vi "OpenConfigFile.vi"(8 "error in (no error)":errorcluster, 11 "GRMActor in":refnum<class "GenericController.lvclass">) -> (0 "error out":errorcluster, 2 "refnum":T1, 3 "GRMActor out":refnum<class "GenericController.lvclass">)   [LabVIEW 2020, in "GenericController.lvlib" / "GenericController.lvclass"]
uses:
  GenericController.lvclass
  <vilib>/Utility/config.llb/Config Data RefNum.ctl
  GenericController.lvclass/GenericController.ctl
  <vilib>/Utility/config.llb/NI_LVConfig.lvlib
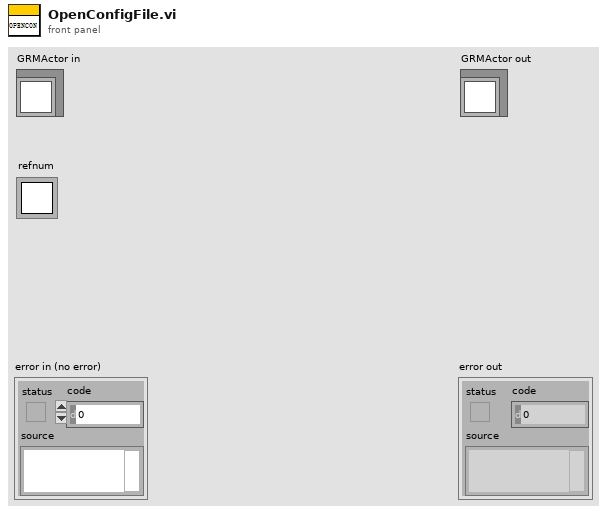
[diagram p1: front panel]
types:
  T1 = typedef "NI_LVConfig.lvlib/Config Data RefNum.ctl" = refnum<k1>
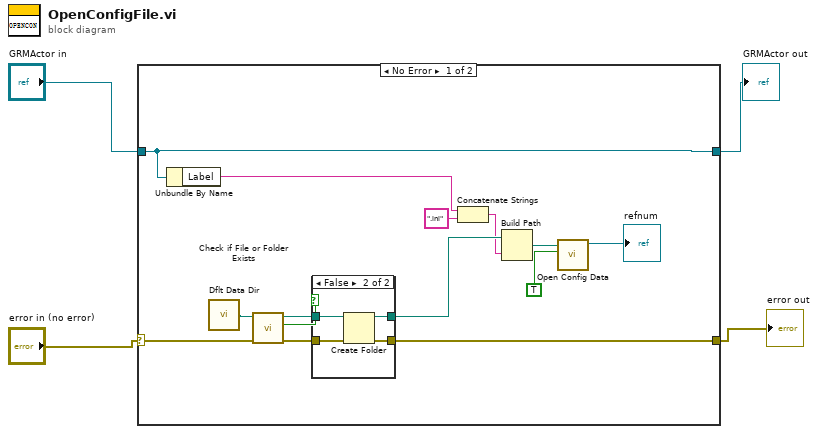
[diagram p0: block diagram]
diagram:
  n1 = case shown="No Error" "error in (no error)" {
    selector: "error in (no error)" -> [w18 w26]
    tunnel: [w17 w26] -> w1
    tunnel: [w15 w25] -> w2
    tunnel: "GRMActor in" -> [w15 w25]
    frame No Error {
      n2 = Unbundle By Name(w15) -> ("Label"=w16:string)
      n3 = call <vilib>:"Dflt Data Dir.vi"() -> ("App:Default Data Directory"=w10:path)
      n4 = call <vilib>:"Check if File or Folder Exists.vi"("error in (no error)"=w18, "path"=w10) -> ("error out"=w12:errorcluster, "file or folder exists?"=w11:bool, "dup path"=w13:path)  [unwired: 7 in]
      n5 = case shown="False" w11 {
        tunnel: w12 -> [w19 w24]
        tunnel: w13 -> [w20 w23]
        tunnel: [w19 w22] -> w17
        tunnel: [w20 w21] -> w9
        frame True {
        }
        frame False {
          n6 = Create Folder(path (use dialog)=w23, error in=w24) -> (created path=w21:path, error out=w22:errorcluster)  [unwired: 1 in, 1 out]
        }
      }
      n7 = Concatenate Strings(w16, ".ini" ("string")) -> (w7:string)
      n8 = Build Path(base path=w9, name or relative path=w7) -> (appended path=w5:path)
      n9 = call <vilib>:"Open Config Data.vi"("create file if necessary (T)"=TRUE, "configuration file path"=w5) -> ("refnum"=→"refnum":T1)  [unwired: 7 in, 2 out]
    }
    frame Error {
    }
  }
  "error out" <- w1
  "GRMActor out" <- w2
